vi "Drive Controller.vi"(8 "error in":errorcluster) -> ()   [LabVIEW 2018]
doc: "This VI executes continuously carrying out the current operation and responding to updates or new operation requests. It will often contain the timing or control code that is difficult to place directly in TeleOp. This VI generally opens all sensors and motors and isolates the rest of the robot code from knowing implementation details of how the operations are carried out."
uses:
  <vilib>/Rock Robotics/WPI/Framework/Completion Status.ctl
  Drive Setpoints.ctl
  Drive Operations.ctl
  <vilib>/Rock Robotics/WPI/ThirdParty/Phoenix-LabVIEW/Motor Controller/Controls/CTRE_Phoenix_MotorControl_NeutralMode.ctl
  <vilib>/Rock Robotics/WPI/ThirdParty/Phoenix-LabVIEW/Motor Controller/Controls/CTRE_Phoenix_MotorControl_FeedbackDevice.ctl
  <vilib>/Rock Robotics/WPI/ThirdParty/Phoenix-LabVIEW/Motor Controller/Controls/CTRE_Phoenix_MotorControl_ControlMode.ctl
  <vilib>/Rock Robotics/WPI/ThirdParty/Phoenix-LabVIEW/Pigeon IMU/CTRE_PigeonIMU_Open_TalonSRX.vi
  <vilib>/Rock Robotics/WPI/ThirdParty/Phoenix-LabVIEW/Motor Controller/Get/CTRE_Phoenix_MotorController_GetSelectedSensorData.vi
  Drive Published Globals.vi
  <vilib>/Rock Robotics/Network Tables/NT Write Number.vi
  <vilib>/Rock Robotics/WPI/ThirdParty/Phoenix-LabVIEW/Motor Controller/Get/CTRE_Phoenix_MotorController_GetVoltage.vi
  <vilib>/Rock Robotics/Network Tables/NT Write Numeric Array.vi
  Support Code/Global Constants.vi
panel:
  in  "Disable Logging":bool=TRUE
  in  "PID Turn":T1={"proportional gain (Kc)"=0.015, "integral time (Ti, min)"=0.0, "derivative time (Td, min)"=0.0}
  out "Encoders":T2(graph)
  out "Left Encoder":dbl=-1185.6884765625
  out "Right Encoder":dbl=-1185.6884765625
  out "gyro":dbl=106.72
  out "Gyro":dbl(graph)=85.48
  in  "Interactive Values":T3={"Operation"=enum."Auto Turn", "Left Setpoint"=0.0, "Right Setpoint"=0.0, "Duration"=0.0, "Distance"=0.0, "Target Angle"=90.0, "Speed"=0.0}
  in  "Buttons":cluster{"Execute Cmd":bool, "Abort Cmd":bool}
  out "Command Timing":cluster{"Start Time (ms)":u32, "Iterations":i32}={"Start Time (ms)"=2214017, "Iterations"=0}
  out "Status":T5
  out "Setpoints":T6(graph)
  out "Current\nCmd":string="Started at  17:19:58.001\nDefault: Reserve,  L 0.0, R 0.0, D 0.000000, Dist 0.0, A 0.0, S 0.000000"
  # "Interactive Command: You may fill in the settings for a command\nand schedule it with the Execute button. You can observe and abort\nany command while fine tuning the code for the controller."
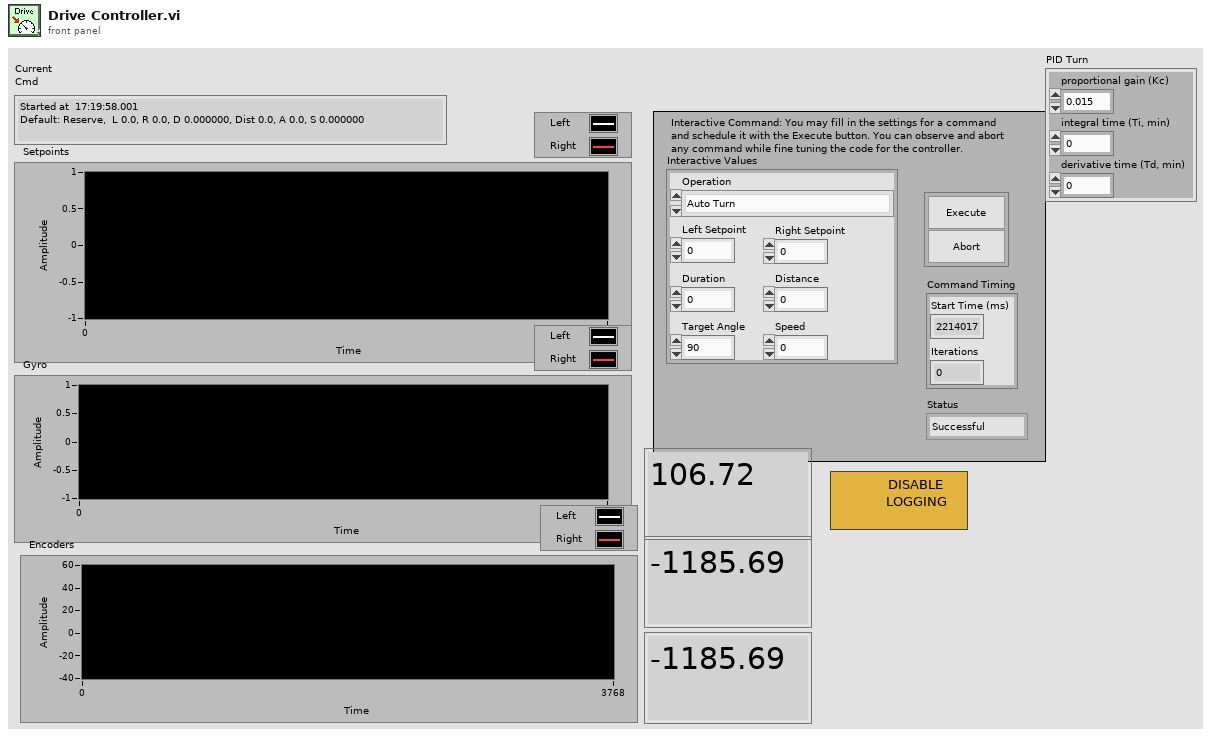
[diagram p1: front panel]
types:
  T1 = cluster{"proportional gain (Kc)":dbl, "integral time (Ti, min)":dbl, "derivative time (Td, min)":dbl}
  T2 = cluster{"Scaled Units (in.)":dbl, "Scaled Units (in.)":dbl}
  T3 = typedef "Drive Setpoints.ctl" = cluster{"Operation":T4, "Left Setpoint":dbl, "Right Setpoint":dbl, "Duration":dbl, "Distance":dbl, "Target Angle":dbl, "Speed":dbl}
  T4 = typedef "Drive Operations.ctl" = enum16{"Reserve", "Read Current", "Immediate", "Drive for Time", "Drive for Distance", "Drive Distance Line", "Drive to Angle Relative", "Drive to Angle", "Run Motion Profile", "Auto Turn", "Reset Encoders", "Reset Gyro"}
  T5 = typedef "Completion Status.ctl" = enum16{"Successful", "Aborted", "Incomplete"}
  T6 = cluster{"Left Setpoint":dbl, "Right Setpoint":dbl}
  T7 = typedef "CTRE_Phoenix_MotorControl_FeedbackDevice.ctl" = i8
  T8 = typedef "CTRE_Phoenix_MotorControl_NeutralMode.ctl" = enum8{"EEPROMSetting", "Override to Coast", "Override to Brake"}
  T9 = typedef "CTRE_Phoenix_MotorControl_ControlMode.ctl" = u16
  T10 = typedef "WPI_MotorControlDeviceRef.ctl" = cluster{"DeviceStatus":errorcluster, "Type":T11, "PWM":cluster{"PWM Channel":T12, "DeadBand":T13}, "CAN":cluster{"Device Number":u8, "SetOutput VI Ref":variant, "GetOutput VI Ref":variant, "Enable VI Ref":variant, "Disable VI Ref":variant, "Data":variant}, "Invert":bool, "DIO PWM":cluster{"PWM \"Enable\" Channel":T12, "DIOChannel":T14, "PWM Rate":dbl}}
  T11 = typedef "WPI_MotorControlType.ctl" = enum16{"PWM", "CAN", "DIO PWM"}
  T12 = typedef "FPGA_DIOPWMChannel.ctl" = enum8{"PWM 0", "PWM 1", "PWM 2", "PWM 3", "PWM 4", "PWM 5", "PWM 6", "PWM 7", "PWM 8", "PWM 9", "PWM MXP 0", "PWM MXP 1", "PWM MXP 2", "PWM MXP 3", "PWM MXP 4", "PWM MXP 5", "PWM MXP 6", "PWM MXP 7", "PWM MXP 8", "PWM MXP 9", "Invalid"}
  T13 = typedef "WPI_PWMDeadband.ctl" = cluster{"Name":string, "maxPositivePwm":i32, "minPositivePwm":i32, "centerPwm":i32, "maxNegativePwm":i32, "minNegativePwm":i32, "angularRange":u16}
  T14 = typedef "FPGA_DIOChannel.ctl" = enum8{"DIO 0", "DIO 1", "DIO 2", "DIO 3", "DIO 4", "DIO 5", "DIO 6", "DIO 7", "DIO 8", "DIO 9", "DIO MXP 0", "DIO MXP 1", "DIO MXP 2", "DIO MXP 3", "DIO MXP 4", "DIO MXP 5", "DIO MXP 6", "DIO MXP 7", "DIO MXP 8", "DIO MXP 9", "DIO MXP 10", "DIO MXP 11", "DIO MXP 12", "DIO MXP 13", "DIO MXP 14", "DIO MXP 15", "SPI Port CS1", "SPI Port CS2", "SPI Port CS3", "SPI Port MISO", "SPI Port MOSI", "Invalid"}
  T15 = typedef "CTRE_PigeonIMU_DeviceRef.ctl" = cluster{"DeviceStatus":errorcluster, "Device Number":u8, "Type":T16, "Device ID":u32, "Handle":u64, "UsageFrame":u32, "Library Path":path}
  T16 = typedef "CTRE_PigeonIMU_ConnectionType.ctl" = u32
  T17 = typedef "Command Status Info.ctl" = cluster{"Name":string, "Status":T5, "notifier out":T18}
  T18 = typedef "Completion Notifier.ctl" = refnum<notifier>
  T19 = cluster{"SubSystem Data":T3, cluster{"Start Time (ms)":u32, "Iterations":i32}, cluster{"Command Info":T17, "Description":string, "Default Command":T3, "queue out":refnum<queue>, "Subsystem Name":string}}
  T20 = typedef "WPI_SwitchDevRef.ctl" = cluster{"DevStatus":errorcluster, "DIO Channel":T14, "CntIndex":T21, "Normally Closed":bool}
  T21 = typedef "FPGA_CounterCtrSystemIndex.ctl" = enum8{"Ctr 0", "Ctr 1", "Ctr 2", "Ctr 3", "Ctr 4", "Ctr 5", "Ctr 6", "Ctr 7", "Invalid"}
  T22 = enum16{"FollowerType_PercentOutput", "FollowerType_AuxOutput1"}
  T23 = enum16{"DemandType_Neutral", "DemandType_AuxPID", "DemandType_ArbitraryFeedForward"}
  T24 = cluster{"SubSystem Data":T3, cluster{"Start Time (ms)":u32, "Iterations":i32}, "Default Command Arguments":cluster{"Command Info":T17, "Description":string, "Default Command":T3, "queue out":refnum<queue>, "Subsystem Name":string}}
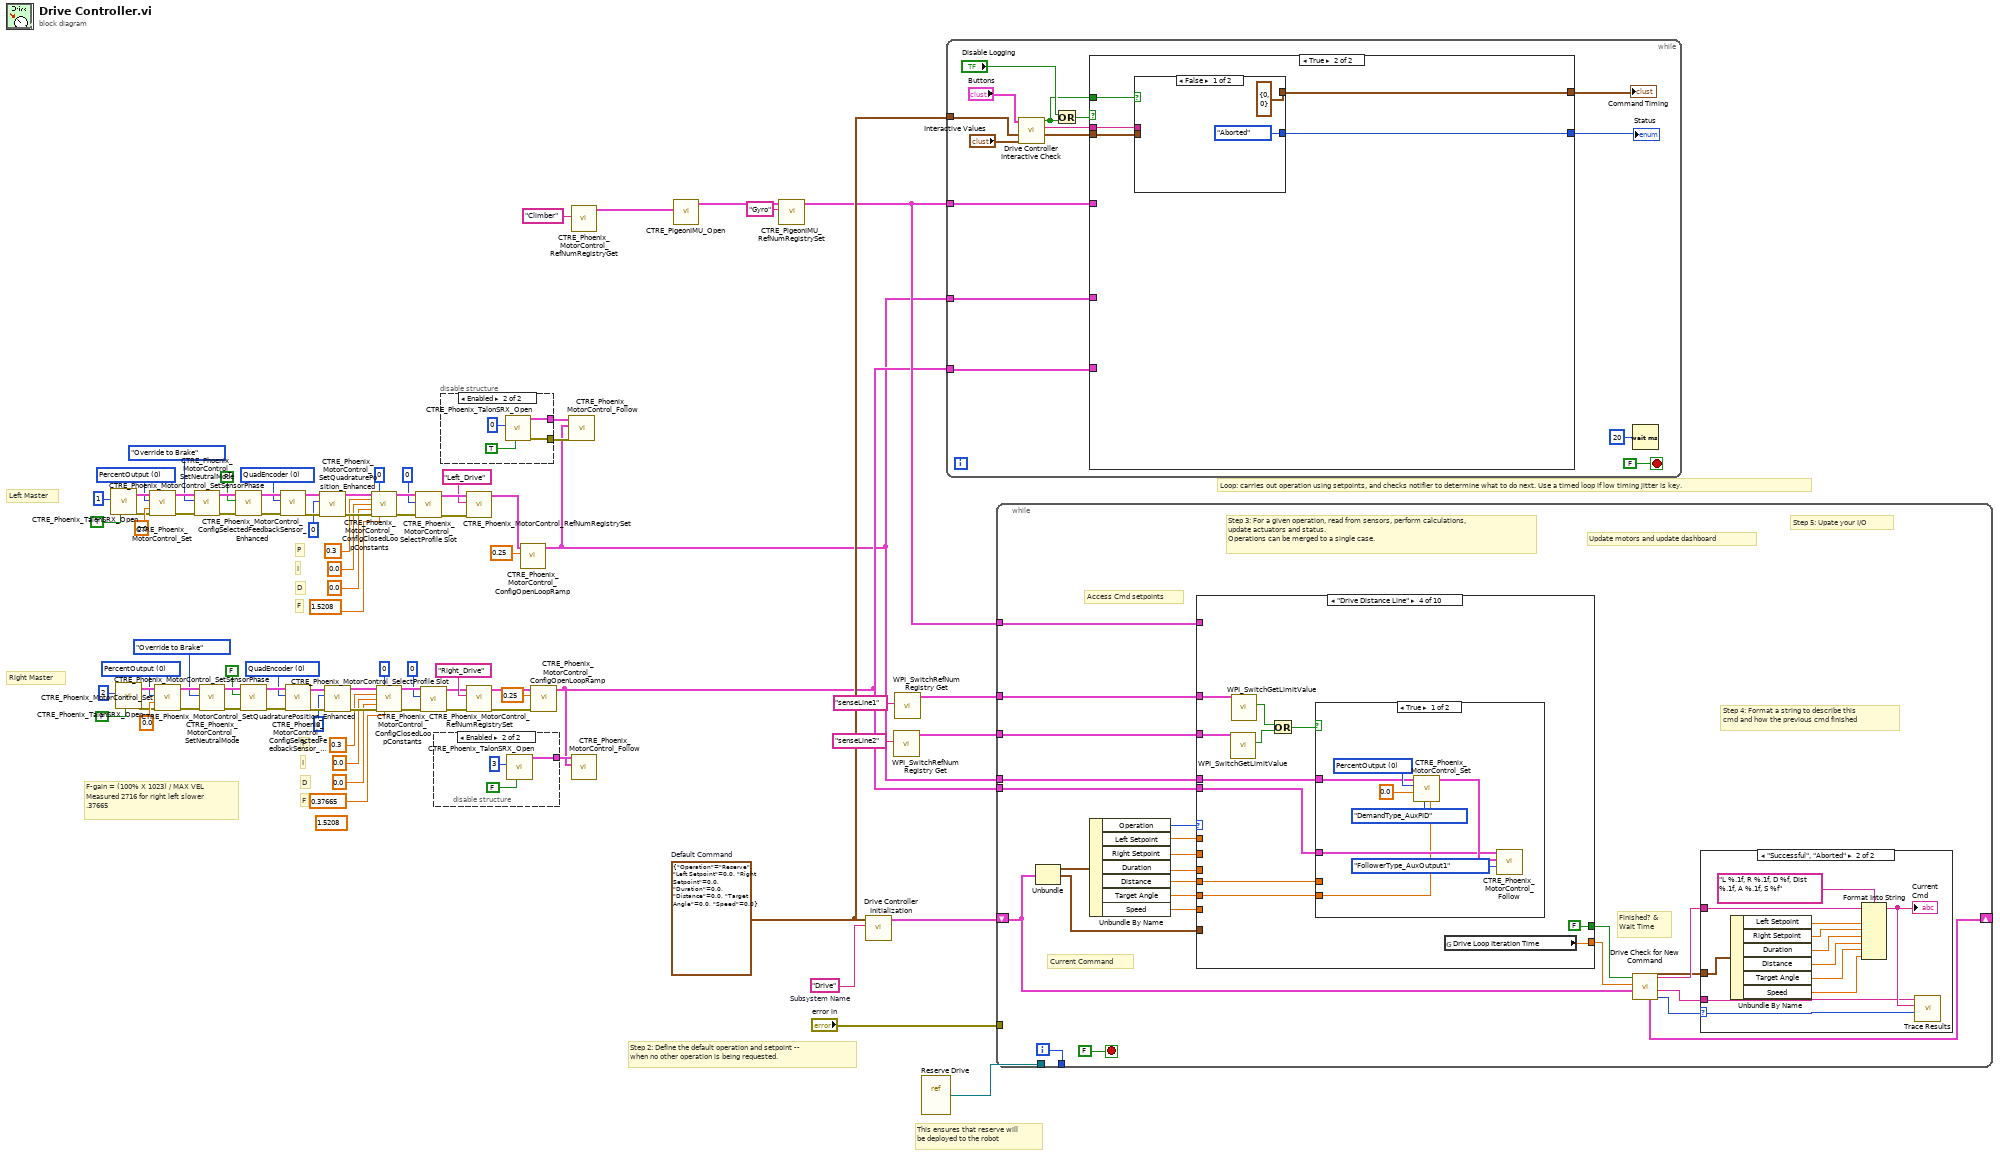
[diagram p0: block diagram]
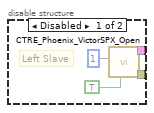
[diagram p2: hidden frame]
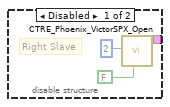
[diagram p3: hidden frame]
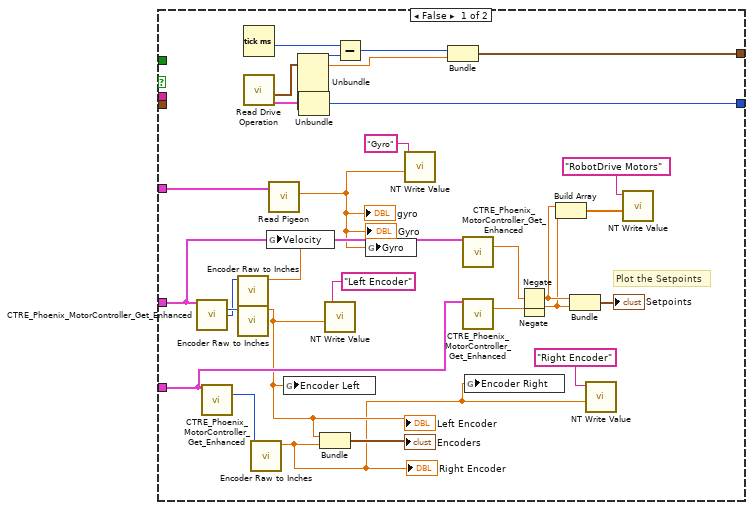
[diagram p4: hidden frame]
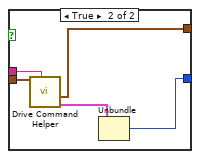
[diagram p5: hidden frame]
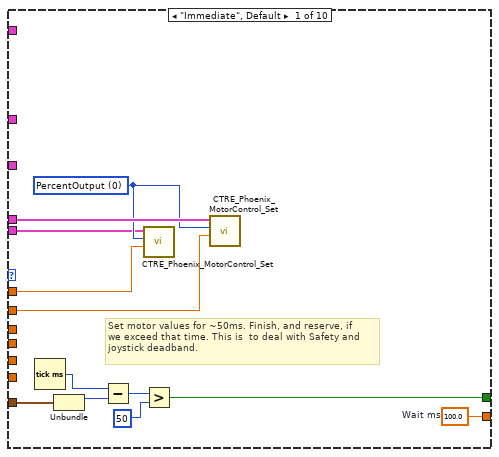
[diagram p7: hidden frame]
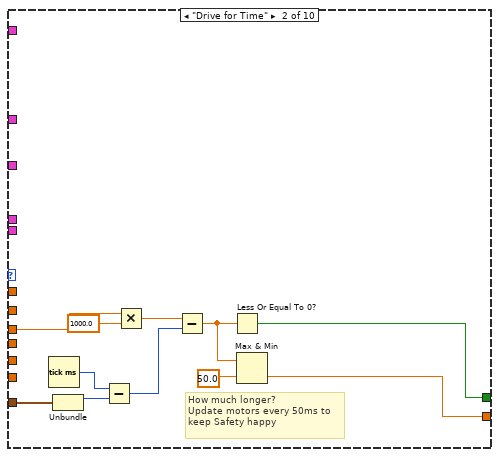
[diagram p8: hidden frame]
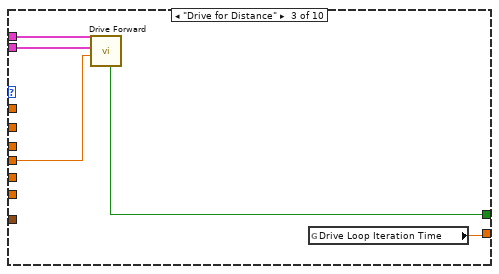
[diagram p9: hidden frame]
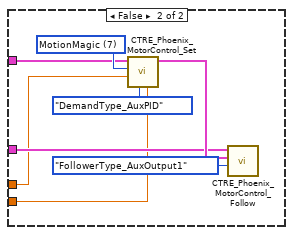
[diagram p10: hidden frame]
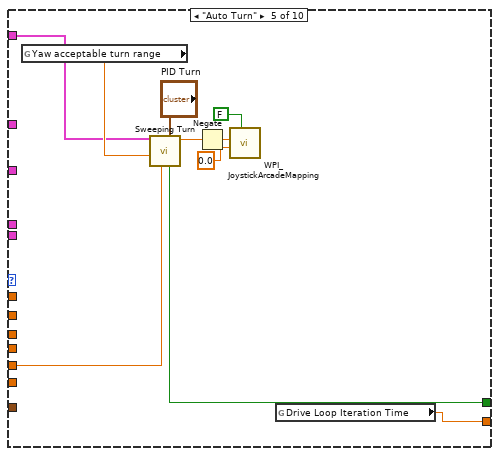
[diagram p11: hidden frame]
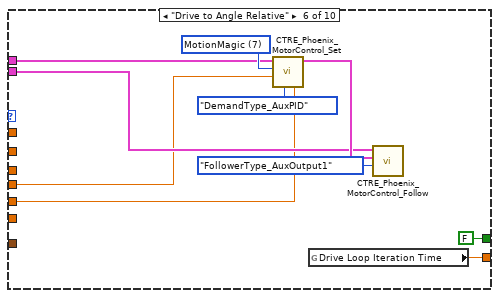
[diagram p12: hidden frame]
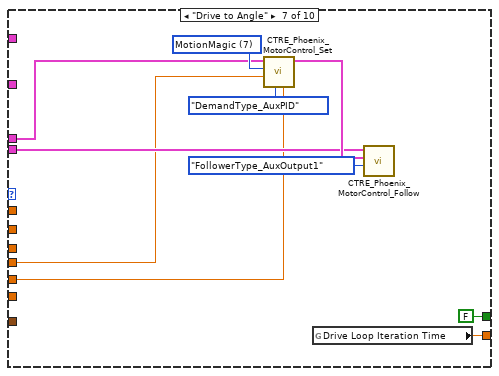
[diagram p13: hidden frame]
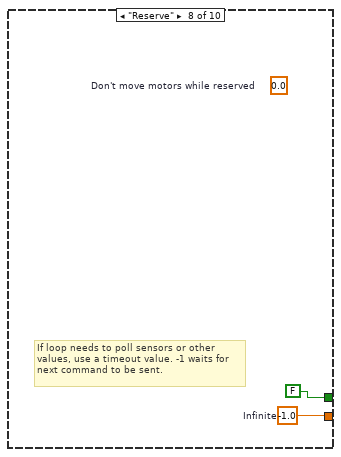
[diagram p14: hidden frame]
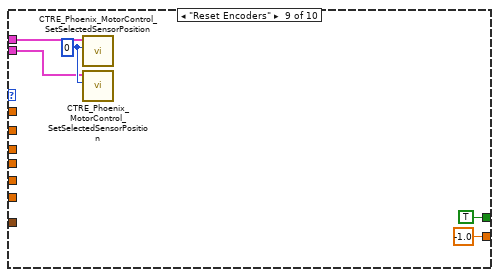
[diagram p15: hidden frame]
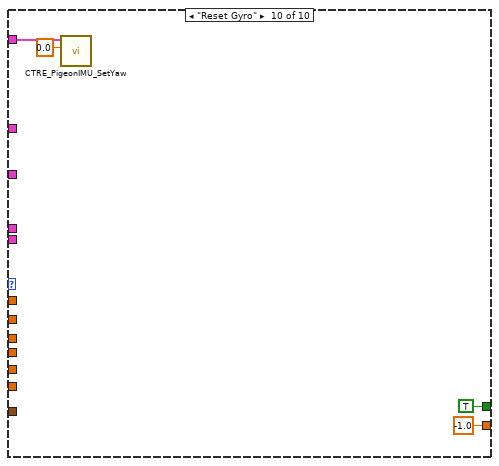
[diagram p16: hidden frame]
diagram:
  (unwired) 1.5208 ("F")
  w38 = T7 0 items=["None"=-1, "QuadEncoder"=0, "Analog"=2, "Tachometer"=4, "Pulse Width Encoded Position"=8, "Sensor Sum (S0 + S1)"=9, "Sensor Difference (D0 - D1)"=10, "Remote Source 0"=11, "Remote Source 1"=12, "Software Emulated"=15] ("Feedback Device")
  w49 = T9 0 items=["PercentOutput"=0, "Position"=1, "Velocity"=2, "Current"=3, "Follower"=5, "MotionProfile"=6, "MotionMagic"=7, "MotionMagicArc"=8, "MotionProfileArc"=10, "Disabled"=15] ("Control Mode")
  w65 = T7 0 items=["None"=-1, "QuadEncoder"=0, "Analog"=2, "Tachometer"=4, "Pulse Width Encoded Position"=8, "Sensor Sum (S0 + S1)"=9, "Sensor Difference (D0 - D1)"=10, "Remote Source 0"=11, "Remote Source 1"=12, "Software Emulated"=15] ("Feedback Device")
  w76 = T9 0 items=["PercentOutput"=0, "Position"=1, "Velocity"=2, "Current"=3, "Follower"=5, "MotionProfile"=6, "MotionMagic"=7, "MotionMagicArc"=8, "MotionProfileArc"=10, "Disabled"=15] ("Control Mode")
  w82 = T3 {"Operation"=enum."Reserve", "Left Setpoint"=0.0, "Right Setpoint"=0.0, "Duration"=0.0, "Distance"=0.0, "Target Angle"=0.0, "Speed"=0.0}  # Default Command
  w86 = "Drive"  # Subsystem Name
  # "F-gain = (100% X 1023) / MAX VEL\nMeasured 2716 for right left slower\n.37665"
  # "Right Master"
  # "Left Master"
  # "F"
  # "D"
  # "I"
  # "P"
  # "F"
  # "D"
  # "I"
  # "P"
  # "This ensures that reserve will\nbe deployed to the robot"
  # "Step 2: Define the default operation and setpoint --\nwhen no other operation is being requested."
  # "Loop: carries out operation using setpoints, and checks notifier to determine what to do next. Use a timed loop if low timing jitter is key."
  n1 = call <vilib>:"CTRE_Phoenix_TalonSRX_Open.vi"("Invert"=TRUE, "Device Number"=u8 1) -> ("error out"=w69:errorcluster, "CAN Talon SRX Ref"=w77:T10)  [unwired: 8 in]
  n2 = call <vilib>:"CTRE_Phoenix_TalonSRX_Open.vi"("Invert"=FALSE, "Device Number"=u8 2) -> ("error out"=w42:errorcluster, "CAN Talon SRX Ref"=w50:T10)  [unwired: 8 in]
  n3 = call <vilib>:"CTRE_Phoenix_MotorControl_Set.vi"("error in (no error)"=w69, "Output"=0.0, "Control Mode"=w76, "PhoenixMotorControlDevRef"=w77) -> ("error out"=w70:errorcluster, "PhoenixMotorControlDevRef"=w74:T10)  [unwired: 6 in]
  n4 = call <vilib>:"CTRE_Phoenix_MotorControl_Set.vi"("error in (no error)"=w42, "Output"=0.0, "Control Mode"=w49, "PhoenixMotorControlDevRef"=w50) -> ("error out"=w43:errorcluster, "PhoenixMotorControlDevRef"=w47:T10)  [unwired: 6 in]
  n5 = call <vilib>:"CTRE_Phoenix_MotorControl_SetNeutralMode.vi"("error in (no error)"=w70, "Motor Control Neutral Mode"=CTRE_Phoenix_MotorControl_NeutralMode."Override to Brake", "PhoenixMotorControlDevRef"=w74) -> ("error out"=w72:errorcluster, "PhoenixMotorControlDevRef"=w71:T10)  [unwired: 7 in]
  n6 = call <vilib>:"CTRE_Phoenix_MotorControl_SetNeutralMode.vi"("error in (no error)"=w43, "Motor Control Neutral Mode"=CTRE_Phoenix_MotorControl_NeutralMode."Override to Brake", "PhoenixMotorControlDevRef"=w47) -> ("error out"=w45:errorcluster, "PhoenixMotorControlDevRef"=w44:T10)  [unwired: 7 in]
  n7 = call <vilib>:"CTRE_Phoenix_MotorControl_SetSensorPhase.vi"("error in (no error)"=w72, "PhaseSensor"=FALSE, "PhoenixMotorControlDevRef"=w71) -> ("error out"=w67:errorcluster, "PhoenixMotorControlDevRef"=w66:T10)  [unwired: 7 in]
  n8 = call <vilib>:"CTRE_Phoenix_MotorControl_SetSensorPhase.vi"("error in (no error)"=w45, "PhaseSensor"=FALSE, "PhoenixMotorControlDevRef"=w44) -> ("error out"=w40:errorcluster, "PhoenixMotorControlDevRef"=w39:T10)  [unwired: 7 in]
  n9 = call <vilib>:"CTRE_Phoenix_MotorControl_ConfigSelectedFeedbackSensor_Enhanced.vi"("error in (no error)"=w67, "Feedback Device"=w65, "PhoenixMotorControlDevRef"=w66) -> ("error out"=w63:errorcluster, "PhoenixMotorControlDevRef"=w64:T10)  [unwired: 7 in]
  n10 = call <vilib>:"CTRE_Phoenix_MotorControl_ConfigSelectedFeedbackSensor_Enhanced.vi"("error in (no error)"=w40, "Feedback Device"=w38, "PhoenixMotorControlDevRef"=w39) -> ("error out"=w36:errorcluster, "PhoenixMotorControlDevRef"=w37:T10)  [unwired: 7 in]
  n11 = call <vilib>:"CTRE_Phoenix_MotorControl_SetQuadraturePosition_Enhanced.vi"("error in (no error)"=w63, "New Position"=0, "PhoenixMotorControlDevRef"=w64) -> ("error out"=w60:errorcluster, "PhoenixMotorControlDevRef"=w61:T10)  [unwired: 7 in]
  n12 = call <vilib>:"CTRE_Phoenix_MotorControl_SetQuadraturePosition_Enhanced.vi"("error in (no error)"=w36, "New Position"=0, "PhoenixMotorControlDevRef"=w37) -> ("error out"=w33:errorcluster, "PhoenixMotorControlDevRef"=w34:T10)  [unwired: 7 in]
  n13 = call <vilib>:"CTRE_Phoenix_MotorControl_ConfigClosedLoopConstants.vi"("PhoenixMotorControlDevRef"=w61, "slotIdx"=0, "P"=0.3, "I"=0.0, "D"=0.0, "error in (no error)"=w60, "F"=1.5208) -> ("PhoenixMotorControlDevRef"=w53:T10, "error out"=w54:errorcluster)  [unwired: 7 in]
  n14 = call <vilib>:"CTRE_Phoenix_MotorControl_ConfigClosedLoopConstants.vi"("PhoenixMotorControlDevRef"=w34, "slotIdx"=0, "P"=0.3, "I"=0.0, "D"=0.0, "error in (no error)"=w33, "F"=0.37665) -> ("PhoenixMotorControlDevRef"=w26:T10, "error out"=w27:errorcluster)  [unwired: 7 in]
  n15 = call <vilib>:"CTRE_Phoenix_MotorControl_SelectProfile Slot.vi"("error in (no error)"=w54, "slotIdx"=0, "PhoenixMotorControlDevRef"=w53) -> ("error out"=w23:errorcluster, "PhoenixMotorControlDevRef"=w22:T10)  [unwired: 7 in]
  n16 = call <vilib>:"CTRE_Phoenix_MotorControl_SelectProfile Slot.vi"("error in (no error)"=w27, "slotIdx"=0, "PhoenixMotorControlDevRef"=w26) -> ("error out"=w19:errorcluster, "PhoenixMotorControlDevRef"=w20:T10)  [unwired: 7 in]
  n17 = disable-structure shown="Enabled" {
    disable-tunnel: [w89 w90] -> w13
    frame Disabled {
      # "Right Slave"
      n18 = call <vilib>:"CTRE_Phoenix_VictorSPX_Open.vi"("Invert"=FALSE, "Device Number"=u8 2) -> ("CAN Talon SRX Ref"=w89:T10)  [unwired: 8 in, 1 out]
    }
    frame Enabled {
      n19 = call <vilib>:"CTRE_Phoenix_TalonSRX_Open.vi"("Invert"=FALSE, "Device Number"=u8 3) -> ("CAN Talon SRX Ref"=w90:T10)  [unwired: 8 in, 1 out]
    }
  }
  n20 = disable-structure shown="Enabled" {
    disable-tunnel: [w95 w97] -> w16
    disable-tunnel: [w94 w98] -> w15
    frame Disabled {
      # "Left Slave"
      n21 = call <vilib>:"CTRE_Phoenix_VictorSPX_Open.vi"("Invert"=TRUE, "Device Number"=u8 1) -> ("error out"=w95:errorcluster, "CAN Talon SRX Ref"=w94:T10)  [unwired: 8 in]
    }
    frame Enabled {
      n22 = call <vilib>:"CTRE_Phoenix_TalonSRX_Open.vi"("Invert"=TRUE, "Device Number"=u8 0) -> ("error out"=w97:errorcluster, "CAN Talon SRX Ref"=w98:T10)  [unwired: 8 in]
    }
  }
  n23 = call <vilib>:"CTRE_Phoenix_MotorControl_RefNumRegistrySet.vi"("error in (no error)"=w23, "refnum name"="Left_Drive", "PhoenixMotorControlDevRef"=w22) -> ("PhoenixMotorControlDevRef"=w5:T10)  [unwired: 7 in, 1 out]
  n24 = call <vilib>:"CTRE_Phoenix_MotorControl_RefNumRegistrySet.vi"("error in (no error)"=w19, "refnum name"="Right_Drive", "PhoenixMotorControlDevRef"=w20) -> ("error out"=w7:errorcluster, "PhoenixMotorControlDevRef"=w10:T10)  [unwired: 7 in]
  n25 = call <vilib>:"CTRE_Phoenix_MotorControl_ConfigOpenLoopRamp.vi"("secondsFromNeutralToFull"=0.25, "PhoenixMotorControlDevRef"=w5) -> ("PhoenixMotorControlDevRef"=w4:T10)  [unwired: 8 in, 1 out]
  n26 = call <vilib>:"CTRE_Phoenix_MotorControl_ConfigOpenLoopRamp.vi"("error in (no error)"=w7, "secondsFromNeutralToFull"=0.25, "PhoenixMotorControlDevRef"=w10) -> ("PhoenixMotorControlDevRef"=w9:T10)  [unwired: 7 in, 1 out]
  n27 = call <vilib>:"CTRE_Phoenix_MotorControl_Follow.vi"("error in (no error)"=w16, "Master Controller to Follow"=w4, "PhoenixMotorControlDevRef"=w15) -> ()  [unwired: 7 in, 2 out]
  n28 = call <vilib>:"CTRE_Phoenix_MotorControl_RefNumRegistryGet.vi"("refnum name"="Climber") -> ("PhoenixMotorControlDevRef"=w12:T10)  [unwired: 9 in, 1 out]
  n29 = call <vilib>:"CTRE_Phoenix_MotorControl_Follow.vi"("Master Controller to Follow"=w9, "PhoenixMotorControlDevRef"=w13) -> ()  [unwired: 8 in, 2 out]
  n30 = call-poly <vilib>:"CTRE_PigeonIMU_Open.vi"("CAN Talon SRX Ref"=w12) -> ("PigeonIMUDevRef"=w81:T15)  [unwired: 9 in, 1 out]
  n31 = call <vilib>:"CTRE_PigeonIMU_RefNumRegistrySet.vi"("refnum name"="Gyro", "PigeonIMUDevRef"=w81) -> ("PigeonIMUDevRef"=w80:T15)  [unwired: 8 in, 1 out]
  n32 = call "Drive Controller Initialization.vi"("Subsystem Name"=w86, "Default Command"=w82) -> ("Current Command"=w84:T19)  [unwired: 9 in]
  n33 = call <vilib>:"WPI_SwitchRefNum Registry Get.vi"("refnum name"="senseLine2") -> ("SwitchDevRef"=w2:T20)  [unwired: 9 in, 1 out]
  n34 = call <vilib>:"WPI_SwitchRefNum Registry Get.vi"("refnum name"="senseLine1") -> ("SwitchDevRef"=w1:T20)  [unwired: 9 in, 1 out]
  n35 = vi-ref "Reserve Drive.vi"() -> (w83:refnum<vi>)
  n36 = while {
    tunnel: w82 -> [w108]
    tunnel: w80 -> [w106]
    tunnel: w4 -> [w105]
    tunnel: w9 -> [w104]
    stop <- FALSE stop-if-true
    n37 = call "Drive Controller Interactive Check.vi"("Interactive Command In"="Interactive Values", "Default Command"=w108, "Buttons"="Buttons") -> ("Interactive Command Out"=w110:T3, "Trace String"=w111:string, "Schedule"=w101:bool)  [unwired: 6 in]
    n38 = Or(x="Disable Logging", y=w101) -> (x .or. y?=w103:bool)
    n39 = case shown="True" w103 {
      tunnel: [w141 w149] -> w112
      tunnel: [w140 w146] -> w113
      tunnel: w111 -> [_ w148]
      tunnel: w110 -> [_ w147]
      tunnel: w106 -> [w136 _]
      tunnel: w105 -> [w135 _]
      tunnel: w104 -> [w134 _]
      tunnel: w101 -> [_ w145]
      frame False {
        # "Plot the Setpoints"
        n40 = call-poly <vilib>:"CTRE_Phoenix_MotorController_Get_Enhanced.vi"("PhoenixMotorControlDevRef"=w135) -> ("Position (Raw Sensor Units)"=w128:i32, "Velocity (Raw Sensor Units per 100 ms)"=w117:i32)  [unwired: 11 in, 2 out]
        n41 = call-poly <vilib>:"CTRE_Phoenix_MotorController_Get_Enhanced.vi"("PhoenixMotorControlDevRef"=w134) -> ("Position (Raw Sensor Units)"=w129:i32)  [unwired: 11 in, 3 out]
        n42 = call "Encoder Raw to Inches.vi"("Raw Sensor Units"=w117) -> ("Scaled Units (in.)"=w116:dbl)  [unwired: 10 in]
        n43 = call "Encoder Raw to Inches.vi"("Raw Sensor Units"=w128) -> ("Scaled Units (in.)"=w120:dbl)  [unwired: 10 in]
        "Left Encoder" <- w120
        n44 = Tick Count (ms)() -> (millisecond timer value=w144:u32)
        n45 = call "Read Drive Operation.vi"() -> ("Command Info"=w138:T17, "SubSystem Data"=w137:T3)  [unwired: 9 in, 1 out]
        n46 = call "Encoder Raw to Inches.vi"("Raw Sensor Units"=w129) -> ("Scaled Units (in.)"=w119:dbl)  [unwired: 10 in]
        "Right Encoder" <- w119
        n47 = global write "Drive Published Globals.vi" "Velocity"(w116) -> ()
        n48 = call "Read Pigeon.vi"("PigeonIMUDevRef"=w136) -> ("Yaw"=w118:dbl)  [unwired: 10 in]
        "gyro" <- w118
        "Gyro" <- w118
        n49 = global write "Drive Published Globals.vi" "Encoder Left"(w120) -> ()
        n50 = Unbundle(w137) -> ("Operation"=w142:T4, "Left Setpoint"=w139:dbl)  [unwired: 5 out]
        n51 = Unbundle(w138) -> ("Status"=w141:T5)  [unwired: 2 out]
        n52 = Bundle("Scaled Units (in.)"=w120, "Scaled Units (in.)"=w119) -> (→"Encoders":T2)  [unwired: 1 in]
        n53 = call-poly <vilib>:"NT Write Value.vi"("Numeric"=w120, "Name"="Left Encoder") -> ()  [unwired: 9 in, 1 out]
        n54 = Subtract(x=w144, y=w142) -> (x-y=w143:u32)
        n55 = global write "Drive Published Globals.vi" "Gyro"(w118) -> ()
        n56 = call-poly <vilib>:"NT Write Value.vi"("Numeric"=w118, "Name"="Gyro") -> ()  [unwired: 9 in, 1 out]
        n57 = Bundle(w143, "Left Setpoint"=w139) -> (w140:cluster{u32, "Left Setpoint":dbl})  [unwired: 1 in]
        n58 = call-poly <vilib>:"CTRE_Phoenix_MotorController_Get_Enhanced.vi"("PhoenixMotorControlDevRef"=w135) -> ("Percent Output"=w126:dbl)  [unwired: 10 in, 4 out]
        n59 = call-poly <vilib>:"CTRE_Phoenix_MotorController_Get_Enhanced.vi"("PhoenixMotorControlDevRef"=w134) -> ("Percent Output"=w125:dbl)  [unwired: 10 in, 4 out]
        n60 = global write "Drive Published Globals.vi" "Encoder Right"(w119) -> ()
        n61 = Negate(x=w126) -> (-x=w122:dbl)
        n62 = Negate(x=w125) -> (-x=w121:dbl)
        n63 = Build Array(w122, w121) -> (w123:dbl[])
        n64 = Bundle(w122, w121) -> (→"Setpoints":cluster{dbl, dbl})  [unwired: 1 in]
        n65 = call-poly <vilib>:"NT Write Value.vi"("Numeric"=w119, "Name"="Right Encoder") -> ()  [unwired: 9 in, 1 out]
        n66 = call-poly <vilib>:"NT Write Value.vi"("Numeric Array"=w123, "Name"="RobotDrive Motors") -> ()  [unwired: 9 in, 1 out]
      }
      frame True {
        n67 = case shown="False" w145 {
          tunnel: [Completion_Status."Aborted" ("Status") w156] -> w149
          tunnel: w148 -> [_ w154]
          tunnel: w147 -> [_ w153]
          tunnel: [cluster{"Start Time (ms)":u32, "Iterations":i32} {"Start Time (ms)"=0, "Iterations"=0} ("Command Timing") w152] -> w146
          frame False {
          }
          frame True {
            n68 = call "Drive Command Helper.vi"("Description"=w154, "SubSystem Data"=w153) -> ("Command Info Out"=w155:T17, "Command Timing"=w152:cluster{"Start Time (ms)":u32, "Iterations":i32})  [unwired: 7 in, 1 out]
            n69 = Unbundle(w155) -> ("Status"=w156:T5)  [unwired: 2 out]
          }
        }
      }
    }
    "Status" <- w112
    "Command Timing" <- w113
    n70 = Wait (ms)(milliseconds to wait=u32 20) -> ()  [unwired: 1 out]
  }
  n71 = while {
    shift-right: [w172] -> _
    shift-left: w84 -> [w165]
    tunnel: [w179] -> _
    tunnel: "error in" -> [_]
    tunnel: w83 -> [_]
    tunnel: w4 -> [w161]
    tunnel: w9 -> [w162]
    tunnel: w80 -> [w160]
    tunnel: w2 -> [w158]
    tunnel: w1 -> [w157]
    i -> [w179]
    stop <- FALSE stop-if-true
    # "Step 5: Upate your I/O"
    # "Step 4: Format a string to describe this\ncmd and how the previous cmd finished"
    # "Current Command"
    # "Update motors and update dashboard"
    # "Access Cmd setpoints"
    # "Finished? &\nWait Time"
    # "Step 3: For a given operation, read from sensors, perform calculations,\nupdate actuators and status.\nOperations can be merged to a single case."
    n72 = Unbundle(w165) -> ("SubSystem Data"=w178:T3, w166:cluster{"Start Time (ms)":u32, "Iterations":i32})  [unwired: 1 out]
    n73 = Unbundle By Name(w178) -> ("Operation"=w177:T4, "Left Setpoint"=w176:dbl, "Right Setpoint"=w175:dbl, "Duration"=w174:dbl, "Distance"=w164:dbl, "Target Angle"=w163:dbl, "Speed"=w159:dbl)
    n74 = case shown="\"Drive Distance Line\"" w177 {
      tunnel: [w204 w206 w216 w231 w257 w267 w268 w279 -1.0 ("Infinite") -1.0 ("Infinite")] -> w171
      tunnel: [w200 w210 w217 FALSE ("ignore previous (F)") w256 FALSE ("ignore previous (F)") FALSE ("ignore previous (F)") FALSE ("ignore previous (F)") TRUE ("ignore previous (F)") TRUE ("ignore previous (F)")] -> w170
      tunnel: w166 -> [w199 w212 _ _ _ _ _ _ _ _]
      tunnel: w176 -> [w194 _ _ _ _ _ _ _ _ _]
      tunnel: w175 -> [w193 _ _ _ _ _ _ _ _ _]
      tunnel: w174 -> [_ w209 _ _ _ _ _ _ _ _]
      tunnel: w164 -> [_ _ w220 w227 _ w259 w270 _ _ _]
      tunnel: w163 -> [_ _ _ w226 w252 w258 w271 _ _ _]
      tunnel: w159 -> [_ _ _ _ _ _ _ _ _ _]
      tunnel: w162 -> [w195 _ w219 w228 _ w261 w272 _ w280 _]
      tunnel: w161 -> [w197 _ w218 w229 _ w262 w273 _ w282 _]
      tunnel: w160 -> [_ _ _ _ w249 _ _ _ _ w286]
      tunnel: w158 -> [_ _ _ w223 _ _ _ _ _ _]
      tunnel: w157 -> [_ _ _ w222 _ _ _ _ _ _]
      frame "Immediate", Default {
        w196 = T9 0 items=["PercentOutput"=0, "Position"=1, "Velocity"=2, "Current"=3, "Follower"=5, "MotionProfile"=6, "MotionMagic"=7, "MotionProfileArc"=10, "Disabled"=15] ("Control Mode")
        w204 = 100.0  # Wait ms
        # "Set motor values for ~50ms. Finish, and reserve, if\nwe exceed that time. This is  to deal with Safety and\njoystick deadband."
        n75 = Tick Count (ms)() -> (millisecond timer value=w198:u32)
        n76 = Unbundle(w199) -> ("Start Time (ms)"=w201:u32)  [unwired: 1 out]
        n77 = Subtract(x=w198, y=w201) -> (x-y=w202:u32)
        n78 = call <vilib>:"CTRE_Phoenix_MotorControl_Set.vi"("Output"=w194, "Control Mode"=w196, "PhoenixMotorControlDevRef"=w195) -> ()  [unwired: 7 in, 2 out]
        n79 = Greater?(x=w202, y=u8 50 ("Left Motor")) -> (0:w200:bool)
        n80 = call <vilib>:"CTRE_Phoenix_MotorControl_Set.vi"("Output"=w193, "Control Mode"=w196, "PhoenixMotorControlDevRef"=w197) -> ()  [unwired: 7 in, 2 out]
      }
      frame "Drive for Time" {
        # "How much longer?\nUpdate motors every 50ms to\nkeep Safety happy"
        n81 = Tick Count (ms)() -> (millisecond timer value=w205:u32)
        n82 = Unbundle(w212) -> ("Start Time (ms)"=w211:u32)  [unwired: 1 out]
        n83 = Subtract(x=w205, y=w211) -> (x-y=w215:u32)
        n84 = Multiply(x=w209, y=1000.0) -> (x*y=w214:dbl)
        n85 = Subtract(x=w214, y=w215) -> (x-y=w208:dbl)
        n86 = Less Or Equal To 0?(x=w208) -> (x <= 0?=w210:bool)
        n87 = Max & Min(x=w208, y=50.0) -> (min(x,y)=w206:dbl)  [unwired: 1 out]
      }
      frame "Drive for Distance" {
        n88 = call "Drive Forward.vi"("Distance"=w220, "rightmotors"=w219, "leftmotors"=w218) -> ("Stop"=w217:bool)  [unwired: 5 in, 3 out]
        n89 = global read "Global Constants.vi" "Drive Loop Iteration Time"() -> (w216:dbl)
      }
      frame "Drive Distance Line" {
        n90 = call <vilib>:"WPI_SwitchGetLimitValue.vi"("SwitchDevRef"=w223) -> ("Switch Pressed"=w224:bool)  [unwired: 8 in, 2 out]
        n91 = call <vilib>:"WPI_SwitchGetLimitValue.vi"("SwitchDevRef"=w222) -> ("Switch Pressed"=w225:bool)  [unwired: 8 in, 2 out]
        n92 = Or(x=w225, y=w224) -> (x .or. y?=w221:bool)
        n93 = case shown="True" w221 {
          tunnel: w229 -> [w235 w243]
          tunnel: w228 -> [w234 w242]
          tunnel: w227 -> [_ w241]
          tunnel: w226 -> [w233 w240]
          frame True {
            w239 = T9 0 items=["PercentOutput"=0, "Position"=1, "Velocity"=2, "Current"=3, "Follower"=5, "MotionProfile"=6, "MotionMagic"=7, "MotionProfileArc"=10, "Disabled"=15] ("Control Mode")
            n94 = call <vilib>:"CTRE_Phoenix_MotorControl_Set.vi"("Demand1"=w233, "DemandType"=T23."DemandType_AuxPID", "Output"=0.0, "Control Mode"=w239, "PhoenixMotorControlDevRef"=w235) -> ("PhoenixMotorControlDevRef"=w237:T10)  [unwired: 5 in, 1 out]
            n95 = call <vilib>:"CTRE_Phoenix_MotorControl_Follow.vi"("FollowerType"=T22."FollowerType_AuxOutput1", "Master Controller to Follow"=w237, "PhoenixMotorControlDevRef"=w234) -> ()  [unwired: 7 in, 2 out]
          }
          frame False {
            w247 = T9 7 items=["PercentOutput"=0, "Position"=1, "Velocity"=2, "Current"=3, "Follower"=5, "MotionProfile"=6, "MotionMagic"=7, "MotionProfileArc"=10, "Disabled"=15] ("Control Mode")
            n96 = call <vilib>:"CTRE_Phoenix_MotorControl_Set.vi"("Demand1"=w240, "DemandType"=T23."DemandType_AuxPID", "Output"=w241, "Control Mode"=w247, "PhoenixMotorControlDevRef"=w243) -> ("PhoenixMotorControlDevRef"=w245:T10)  [unwired: 5 in, 1 out]
            n97 = call <vilib>:"CTRE_Phoenix_MotorControl_Follow.vi"("FollowerType"=T22."FollowerType_AuxOutput1", "Master Controller to Follow"=w245, "PhoenixMotorControlDevRef"=w242) -> ()  [unwired: 7 in, 2 out]
          }
        }
        n98 = global read "Global Constants.vi" "Drive Loop Iteration Time"() -> (w231:dbl)
      }
      frame "Auto Turn" {
        n99 = global read "Global Constants.vi" "Yaw acceptable turn range"() -> (w255:dbl)
        n100 = call "Sweeping Turn.vi"("PID gains"="PID Turn", "Target Yaw"=w252, "Acceptable Range"=w255, "PigeonIMUDevRef"=w249) -> ("Yaw Output"=w254:dbl, "Stop"=w256:bool)  [unwired: 4 in, 2 out]
        n101 = Negate(x=w254) -> (-x=w248:dbl)
        n102 = call <vilib>:"WPI_JoystickArcadeMapping.vi"("Square Inputs"=FALSE, "Y axis value"=0.0 ("Y axis value (Speed)"), "X axis value"=w248) -> ()  [unwired: 7 in, 2 out]
        n103 = global read "Global Constants.vi" "Drive Loop Iteration Time"() -> (w257:dbl)
      }
      frame "Drive to Angle Relative" {
        w266 = T9 7 items=["PercentOutput"=0, "Position"=1, "Velocity"=2, "Current"=3, "Follower"=5, "MotionProfile"=6, "MotionMagic"=7, "MotionProfileArc"=10, "Disabled"=15] ("Control Mode")
        n104 = call <vilib>:"CTRE_Phoenix_MotorControl_Set.vi"("Demand1"=w258, "DemandType"=T23."DemandType_AuxPID", "Output"=w259, "Control Mode"=w266, "PhoenixMotorControlDevRef"=w262) -> ("PhoenixMotorControlDevRef"=w264:T10)  [unwired: 5 in, 1 out]
        n105 = global read "Global Constants.vi" "Drive Loop Iteration Time"() -> (w267:dbl)
        n106 = call <vilib>:"CTRE_Phoenix_MotorControl_Follow.vi"("FollowerType"=T22."FollowerType_AuxOutput1", "Master Controller to Follow"=w264, "PhoenixMotorControlDevRef"=w261) -> ()  [unwired: 7 in, 2 out]
      }
      frame "Drive to Angle" {
        w277 = T9 7 items=["PercentOutput"=0, "Position"=1, "Velocity"=2, "Current"=3, "Follower"=5, "MotionProfile"=6, "MotionMagic"=7, "MotionProfileArc"=10, "Disabled"=15] ("Control Mode")
        n107 = call <vilib>:"CTRE_Phoenix_MotorControl_Set.vi"("Demand1"=w271, "DemandType"=T23."DemandType_AuxPID", "Output"=w270, "Control Mode"=w277, "PhoenixMotorControlDevRef"=w273) -> ("PhoenixMotorControlDevRef"=w275:T10)  [unwired: 5 in, 1 out]
        n108 = global read "Global Constants.vi" "Drive Loop Iteration Time"() -> (w268:dbl)
        n109 = call <vilib>:"CTRE_Phoenix_MotorControl_Follow.vi"("FollowerType"=T22."FollowerType_AuxOutput1", "Master Controller to Follow"=w275, "PhoenixMotorControlDevRef"=w272) -> ()  [unwired: 7 in, 2 out]
      }
      frame "Reserve" {
        (unwired) 0.0  # Don't move motors while reserved
        w279 = -1.0  # Infinite
        # "If loop needs to poll sensors or other\nvalues, use a timeout value. -1 waits for\nnext command to be sent."
      }
      frame "Reset Encoders" {
        w281 = 0 ("New Sensor Position")
        n110 = call <vilib>:"CTRE_Phoenix_MotorControl_SetSelectedSensorPosition.vi"("New Sensor Position"=w281, "PhoenixMotorControlDevRef"=w282) -> ()  [unwired: 8 in, 2 out]
        n111 = call <vilib>:"CTRE_Phoenix_MotorControl_SetSelectedSensorPosition.vi"("New Sensor Position"=w281, "PhoenixMotorControlDevRef"=w280) -> ()  [unwired: 8 in, 2 out]
      }
      frame "Reset Gyro" {
        n112 = call <vilib>:"CTRE_PigeonIMU_SetYaw.vi"("Value"=0.0, "PigeonIMUDevRef"=w286) -> ()  [unwired: 8 in, 2 out]
      }
    }
    n113 = call "Drive Check for New Command.vi"("input cluster"=w165, "Wait time (ms)"=w171, "Finished?"=w170) -> ("Completion"=w173:T5, "Subsystem Name"=w167:string, "Current Command"=w168:T3, "Initial Trace String"=w169:string, "Next Command"=w172:T24)  [unwired: 4 in]
    n114 = case shown="\"Successful\", \"Aborted\"" w173 {
      selector: w173 -> [_ w192]
      tunnel: w169 -> [_ w187]
      tunnel: w168 -> [_ w188]
      tunnel: w167 -> [_ w184]
      frame "Incomplete", Default {
        # "Continuing current command"
      }
      frame "Successful", "Aborted" {
        # "Report and setup for next command"
        n115 = Unbundle By Name(w188) -> ("Left Setpoint"=w190:dbl, "Right Setpoint"=w191:dbl, "Duration"=w185:dbl, "Distance"=w183:dbl, "Target Angle"=w182:dbl, "Speed"=w181:dbl)
        n116 = Format Into String(format string="L %.1f, R %.1f, D %f, Dist %.1f, A %.1f, S %f", initial string=w187, w190, w191, w185, w183, w182, w181) -> (resulting string=w186:string)  [unwired: 1 in, 1 out]
        "Current\nCmd" <- w186
        n117 = call <vilib>:"Trace Results.vi"("Status of previous command"=w192, "Description"=w186, "Subsystem"=w184) -> ()  [unwired: 9 in]
      }
    }
  }
